vi "Main.vi"(8 "error":errorcluster) -> (0 "Error out":errorcluster)   [LabVIEW 2018, in "Serial.lvclass"]
doc: "Use this template to build a simple state machine design pattern. Each state executes code and determines which state to transition to."
uses:
  Serial.lvclass
  Controller/Public Controls/GlobalConfig.ctl
  Serial.lvclass/Serial.ctl
  <vilib>/Instr/_visa.llb/VISA Configure Serial Port (Instr).vi
  Controller/GUI.lvclass
panel:
  out "Double":dbl[](array[numeric])
  out "Raw Read":string[](array[string])
  # "Serial MAIN"
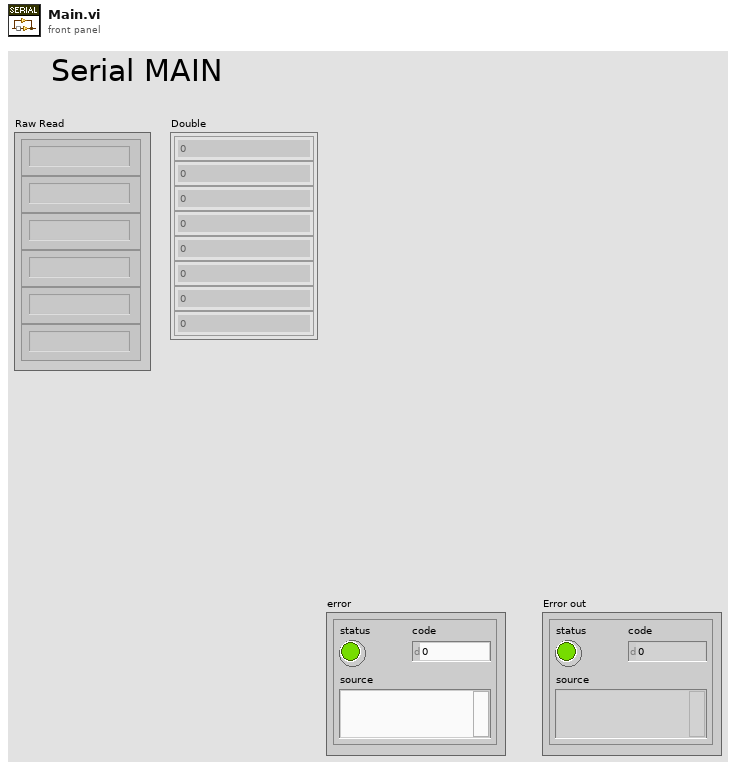
[diagram p1: front panel]
types:
  T1 = typedef "GUI.lvclass/GlobalConfig.ctl" = cluster{"Report Folder Path":path, "PT1_MIN":dbl, "PT1_MAX":dbl, "VENT_PMAX":dbl, "LOP_TARGET":dbl, "LOP_RAMP":dbl, "LOP_LEAK_MAX":dbl, "HIP_TARGET":dbl, "HIP_RAMP":dbl, "HIP_MIN":dbl, "HIP_MAX":dbl, "BLEED_TIME":dbl, "LOP_MAX":dbl, "LOP_MIN":dbl, "PT131Com":refnum<visa-resource-name>, "PT231Com":refnum<visa-resource-name>, "PT331Com":refnum<visa-resource-name>, "PT431Com":refnum<visa-resource-name>, "PT531Com":refnum<visa-resource-name>, "PT631Com":refnum<visa-resource-name>}
  T2 = typedef "Serial.lvclass/State.ctl" = enum16{"Initialize", "LoadConfig", "Read", "Error", "Exit"}
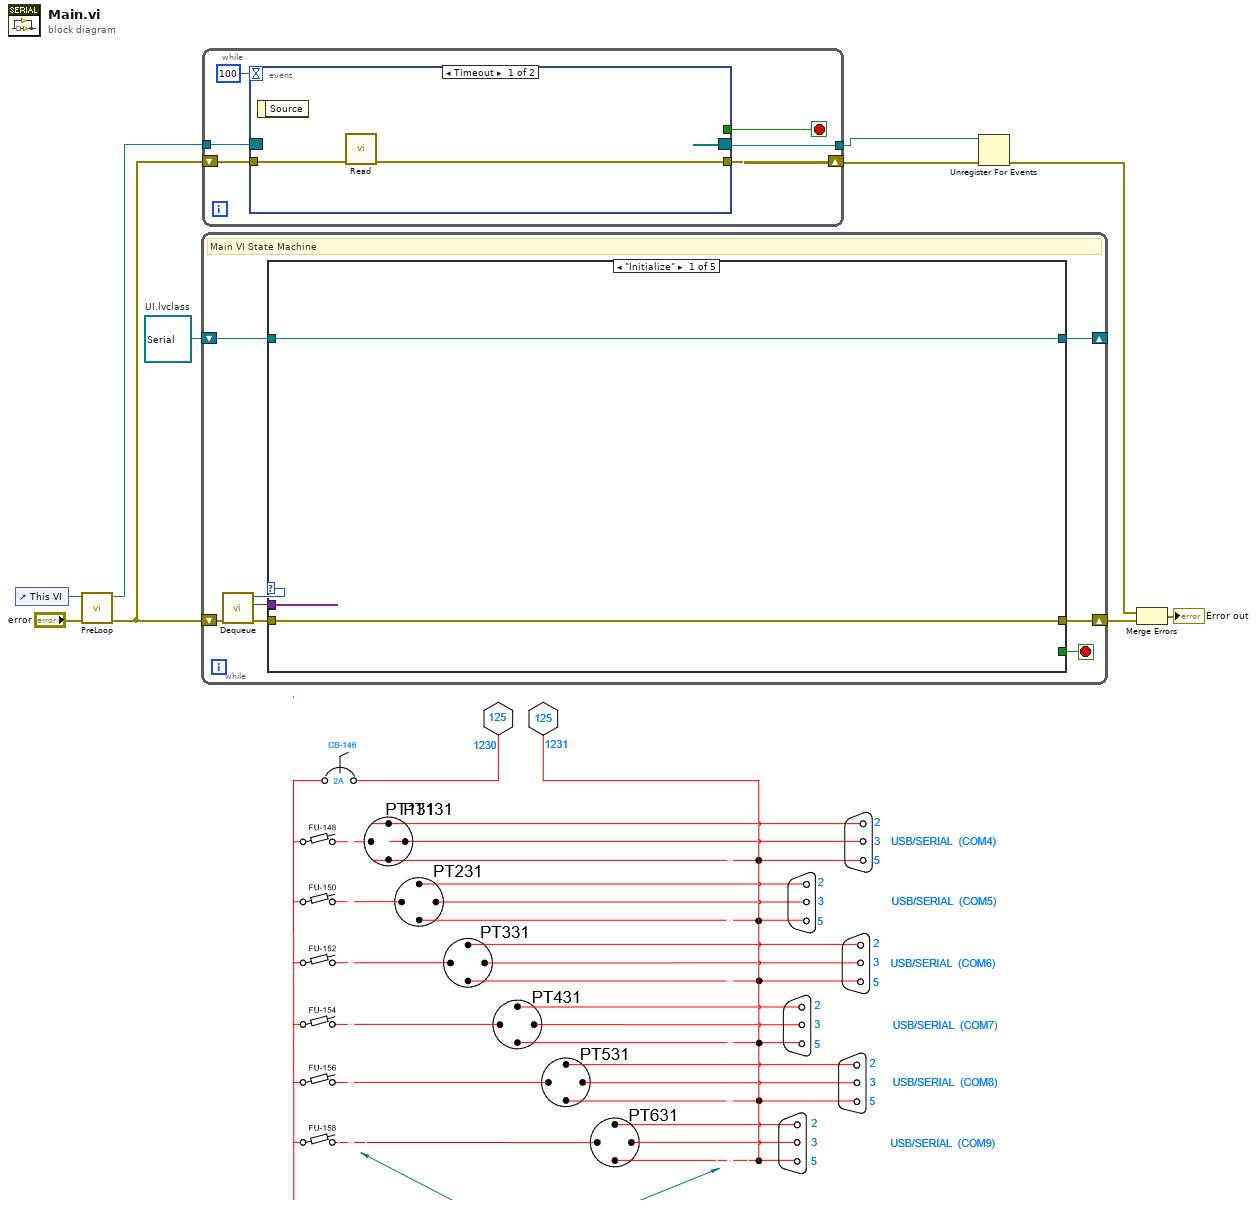
[diagram p0: block diagram]
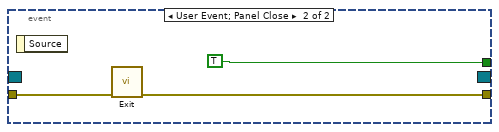
[diagram p2: hidden frame]
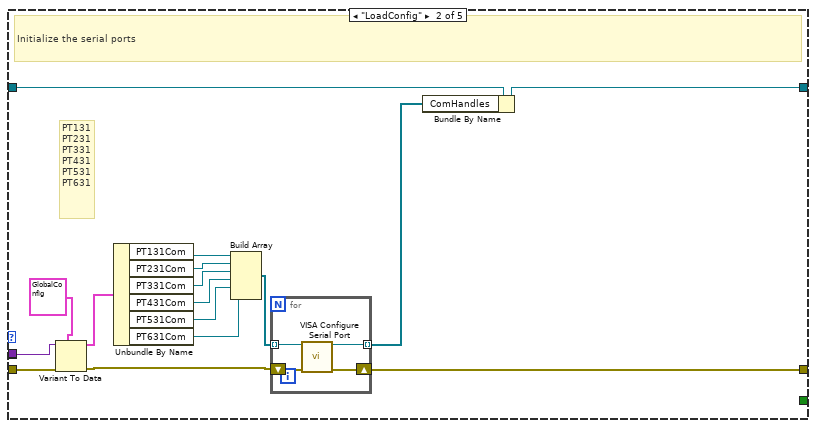
[diagram p3: hidden frame]
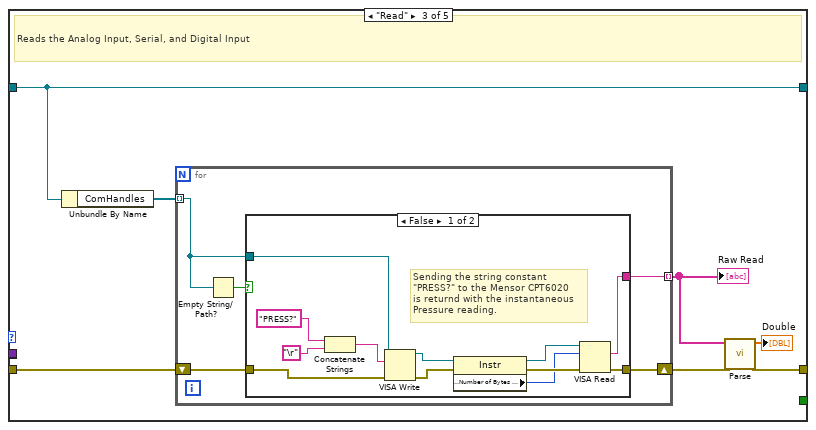
[diagram p4: hidden frame]
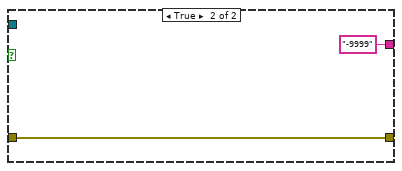
[diagram p5: hidden frame]
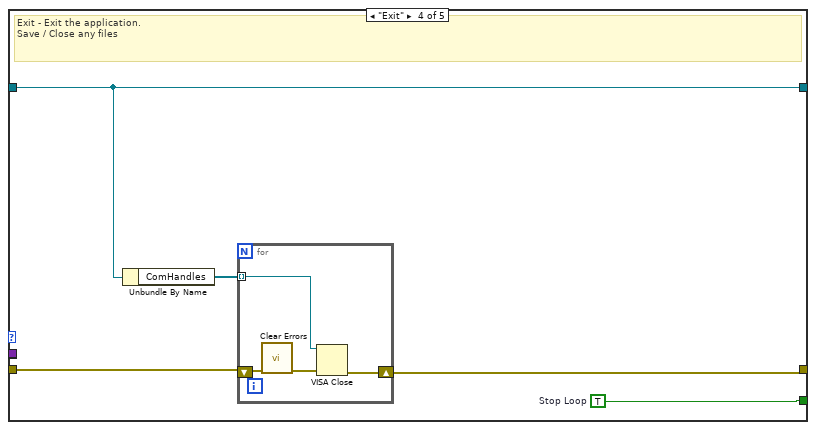
[diagram p6: hidden frame]
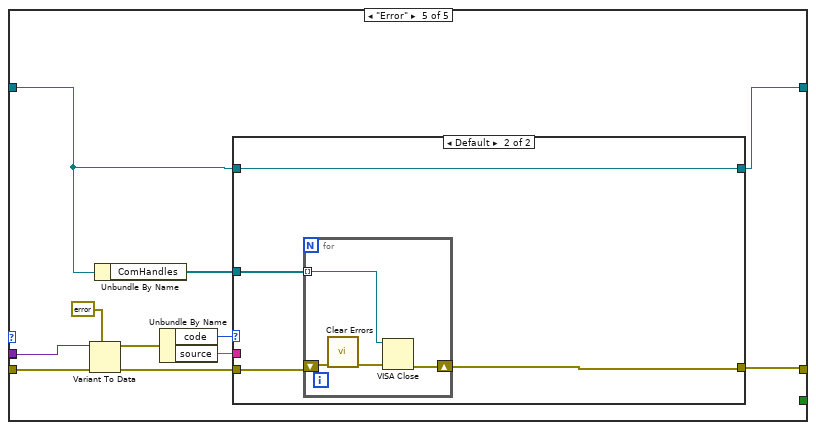
[diagram p7: hidden frame]
diagram:
  w10 = refnum<class "Serial.lvclass"> refnum  # UI.lvclass
  n1 = control-ref of="This VI"() -> (w7:refnum<vi>)
  n2 = call "PreLoop.vi"("error in"="error", "VI Ref"=w7) -> ("error out"=w6:errorcluster, "Event Registration Refnum"=w8:refnum<event-registration>)  [unwired: 8 in]
  n3 = while {
    shift-right: [w18] -> w3
    shift-left: w6 -> [w14]
    shift-right: [w15] -> _
    shift-left: w10 -> [w16]
    stop <- w17 stop-if-true
    # "Main VI State Machine"
    n4 = call "Dequeue.vi"("error in"=w14) -> ("error out"=w13:errorcluster, "Data"=w11:variant, "State"=w12:T2)  [unwired: 8 in]
    n5 = case shown="\"Initialize\"" w12 {
      tunnel: [_ _ _ w71 _] -> w17
      tunnel: w13 -> [w20 w32 w47 w68 w84]
      tunnel: [w20 w35 w42 w67 w80] -> w18
      tunnel: w16 -> [w19 w36 w46 w70 w77]
      tunnel: [w19 w34 w46 w70 w76] -> w15
      tunnel: w11 -> [_ w31 _ _ w83]
      tunnel: w11 -> [_ _ _ _ _]
      frame "Initialize" {
      }
      frame "LoadConfig" {
        # "PT131\nPT231\nPT331\nPT431\nPT531\nPT631"
        # "Initialize the serial ports"
        n6 = Variant To Data(error in=w32, type=T1 {"Report Folder Path"=path "", "PT1_MIN"=0.0, "PT1_MAX"=0.0, "VENT_PMAX"=0.0, "LOP_TARGET"=0.0, "LOP_RAMP"=0.0, "LOP_LEAK_MAX"=0.0, "HIP_TARGET"=0.0, "HIP_RAMP"=0.0, "HIP_MIN"=0.0, "HIP_MAX"=0.0, "BLEED_TIME"=0.0, "LOP_MAX"=0.0, "LOP_MIN"=0.0, "PT131Com"="COM5", "PT231Com"="COM6", "PT331Com"="COM7", "PT431Com"="COM8", "PT531Com"="COM9", "PT631Com"="COM10"} ("Global"), Variant=w31) -> (data=w29:T1, error out=w21:errorcluster)
        n7 = Unbundle By Name(w29) -> ("PT131Com"=w28:refnum<visa-resource-name>, "PT231Com"=w27:refnum<visa-resource-name>, "PT331Com"=w26:refnum<visa-resource-name>, "PT431Com"=w25:refnum<visa-resource-name>, "PT531Com"=w24:refnum<visa-resource-name>, "PT631Com"=w23:refnum<visa-resource-name>)
        n8 = Build Array(w28, w27, w26, w25, w24, w23) -> (w22:refnum<visa-resource-name>[])
        n9 = for {
          shift-right: [w39] -> w35
          shift-left: w21 -> [w40]
          tunnel: w22 -> [w38] mode=indexing
          tunnel: [w37] -> w33 mode=indexing
          n10 = call-poly "VISA Configure Serial Port"("VISA resource name"=w38, "error in (no error)"=w40) -> ("VISA resource name out"=w37:refnum<visa-resource-name>, "error out"=w39:errorcluster)  [unwired: 12 in]
        }
        n11 = Bundle By Name(cluster=w36, "ComHandles"=w33) -> (w34:refnum<class "Serial.lvclass">)
      }
      frame "Read" {
        # "Reads the Analog Input, Serial, and Digital Input"
        n12 = Unbundle By Name(w46) -> ("ComHandles"=w45:refnum<visa-resource-name>[])
        n13 = for {
          shift-right: [w51] -> w44
          shift-left: w47 -> [w52]
          tunnel: w45 -> [w50] mode=indexing
          tunnel: [w49] -> w43 mode=indexing
          n14 = Empty String/Path?(string/path=w50) -> (empty?=w48:bool)
          n15 = case shown="False" w48 {
            tunnel: w52 -> [w57 w66]
            tunnel: [w56 w66] -> w51
            tunnel: w50 -> [w54 _]
            tunnel: [w53 "-9999" ("read buffer")] -> w49
            frame False {
              # "Sending the string constant\n\"PRESS?\" to the Mensor CPT6020\nis returnd with the instantaneous\nPressure reading."
              n16 = Concatenate Strings("PRESS?" ("write buffer"), "\r") -> (w62:string)
              n17 = VISA Write(VISA resource name=w54, write buffer=w62, error in (no error)=w57) -> (VISA resource name out=w58:refnum<visa-resource-name>, error out=w59:errorcluster)  [unwired: 1 out]
              n18 = property class="Instr"(reference=w58, error in=w59) -> (reference out=w64:refnum<visa-resource-name>, error out=w63:errorcluster, "Serial Settings:Number of Bytes at Serial Port"=w55:u32)
              n19 = VISA Read(VISA resource name=w64, byte count=w55, error in (no error)=w63) -> (read buffer=w53:string, error out=w56:errorcluster)  [unwired: 2 out]
            }
            frame True {
            }
          }
        }
        "Raw Read" <- w43
        n20 = call "Parse.vi"("error in (no error)"=w44, "Array"=w43) -> ("error out"=w42:errorcluster, "Double"=→"Double":dbl[])  [unwired: 8 in]
      }
      frame "Exit" {
        w71 = TRUE  # Stop Loop
        # "Exit - Exit the application.\nSave / Close any files"
        n21 = Unbundle By Name(w70) -> ("ComHandles"=w69:refnum<visa-resource-name>[])
        n22 = for {
          tunnel: w69 -> [w72] mode=indexing
          shift-right: [w73] -> w67
          shift-left: w68 -> [w75]
          n23 = call <vilib>:"Clear Errors.vi"("error in (no error)"=w75) -> ("error out"=w74:errorcluster)  [unwired: 5 in, 1 out]
          n24 = VISA Close(VISA resource name=w72, error in (no error)=w74) -> (error out=w73:errorcluster)
        }
      }
      frame "Error" {
        n25 = Variant To Data(error in=w84, type=errorcluster {"status"=FALSE, "code"=0, "source"=""} ("error out"), Variant=w83) -> (data=w85:errorcluster, error out=w81:errorcluster)
        n26 = Unbundle By Name(w77) -> ("ComHandles"=w78:refnum<visa-resource-name>[])
        n27 = Unbundle By Name(w85) -> ("code"=w79:i32, "source"=w82:string)
        n28 = case shown="Default" w79 {
          tunnel: w82 -> [_ _]
          tunnel: w81 -> [w88 w92]
          tunnel: [w88 w89] -> w80
          tunnel: w78 -> [_ w91]
          tunnel: w77 -> [w87 w90]
          tunnel: [w87 w90] -> w76
          frame 1 {
            # "Error talking to other modules. \n\nIgnore. If testing by itself."
          }
          frame Default {
            n29 = for {
              tunnel: w91 -> [w93] mode=indexing
              shift-right: [w94] -> w89
              shift-left: w92 -> [w96]
              n30 = call <vilib>:"Clear Errors.vi"("error in (no error)"=w96) -> ("error out"=w95:errorcluster)  [unwired: 5 in, 1 out]
              n31 = VISA Close(VISA resource name=w93, error in (no error)=w95) -> (error out=w94:errorcluster)
            }
          }
        }
      }
    }
  }
  n32 = while {
    tunnel: w8 -> [w97]
    shift-right: [w100] -> w5
    shift-left: w6 -> [w102]
    tunnel: [w99] -> w4
    stop <- w101 stop-if-true
    n33 = event shown="[0] Timeout" {
      selector: w97 -> [_ _]
      dyn-events: [_ _] -> w99
      timeout: 100 -> [_ _]
      tunnel: w102 -> [w104 w107]
      tunnel: [w103 w106] -> w100
      tunnel: [_ TRUE] -> w101
      event Timeout {
        n34 = event-data() -> ()  [unwired: 1 in, 1 out]
        n35 = call "Read.vi"("error in"=w104) -> ("error out"=w103:errorcluster)  [unwired: 10 in]
      }
      event User Event; Panel Close {
        n36 = event-data() -> ()  [unwired: 1 in, 1 out]
        n37 = call "Exit.vi"("error in"=w107) -> ("error out"=w106:errorcluster)  [unwired: 10 in]
      }
    }
  }
  n38 = Unregister For Events(event registration refnum=w4, error in=w5) -> (error out=w2:errorcluster)
  n39 = Merge Errors(w2, w3) -> (→"Error out":errorcluster)
